vi "Control Channels2512.vi"(8 "error in (no error)":errorcluster, 10 "Values":dbl[](array[numeric]), 11 "IVI Refnum in":refnum<k15>) -> (0 "error Out":errorcluster, 3 "IVI Refnum out":refnum<k15>)   [LabVIEW 2020, in "PXI-2512 Engine.lvlib"]
uses:
  PXI-2512 Engine.lvlib
  <instrlib>/niSwitch/niSwitch.llb/niSwitch Relay Action.ctl
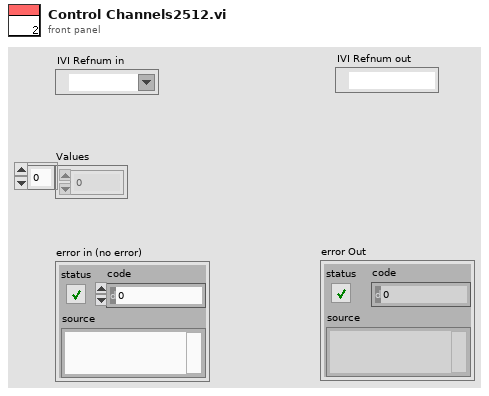
[diagram p1: front panel]
types:
  T1 = enum16{"Default", "DUT Pass Through", "DUT Open", "DUT Pass Through and FB A", "DUT Pass Through and FB B", "DUT FB A", "DUT FB B"}
  T2 = typedef "niSwitch Relay Action.ctl" = i32
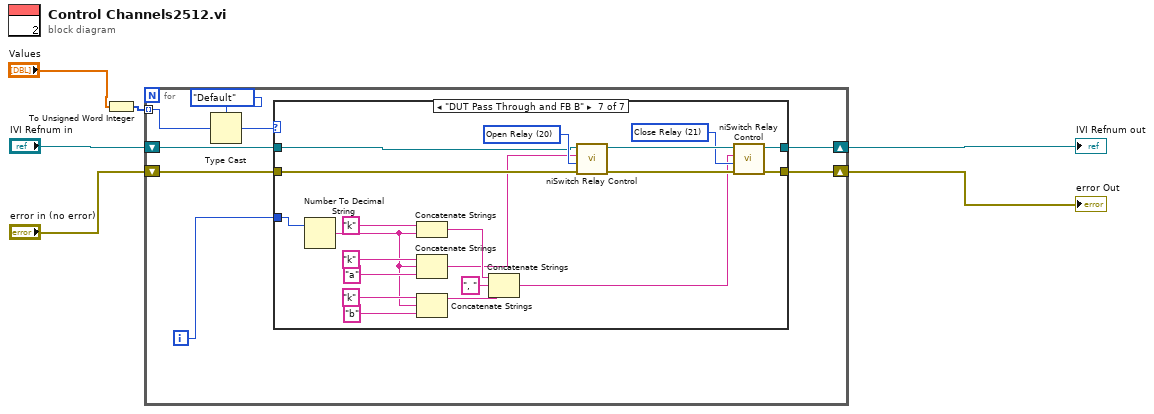
[diagram p0: block diagram]
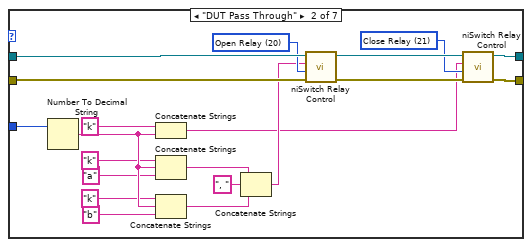
[diagram p3: hidden frame]
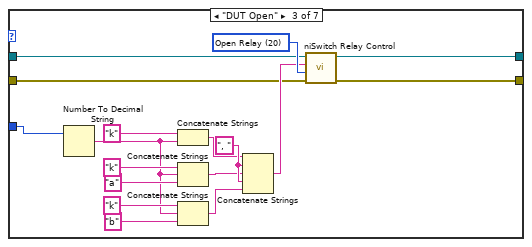
[diagram p4: hidden frame]
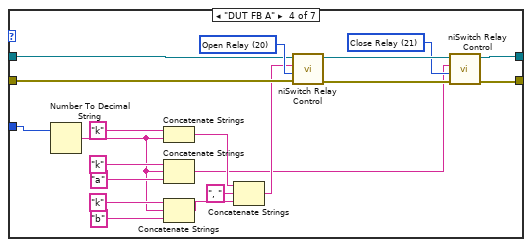
[diagram p5: hidden frame]
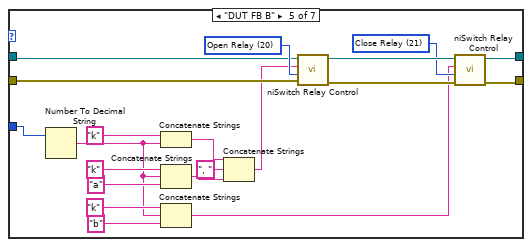
[diagram p6: hidden frame]
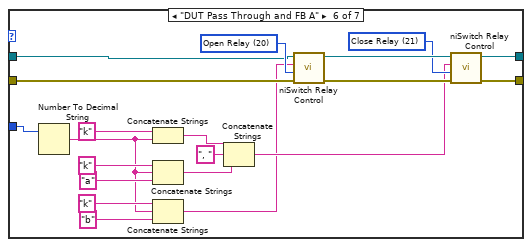
[diagram p7: hidden frame]
diagram:
  n1 = To Unsigned Word Integer(number="Values") -> (unsigned 16bit integer=w5:u16[])
  n2 = for {
    tunnel: w5 -> [w12] mode=indexing
    shift-right: [w10] -> w2
    shift-left: "IVI Refnum in" -> [w14]
    shift-right: [w8] -> w1
    shift-left: "error in (no error)" -> [w9]
    i -> [w7]
    n3 = Type Cast(type=T1."Default", x=w12) -> (*(type *) &x=w11:T1)
    n4 = case shown="\"DUT Pass Through and FB B\"" w11 {
      tunnel: w14 -> [w16 w36 w38 w61 w79 w96 w118]
      tunnel: [w16 w24 w41 w58 w77 w99 w120] -> w10
      tunnel: w9 -> [w15 w22 w37 w60 w78 w97 w117]
      tunnel: [w15 w23 w40 w59 w76 w98 w119] -> w8
      tunnel: w7 -> [_ w26 w43 w55 w84 w104 w114]
      frame "Default", Default {
      }
      frame "DUT Pass Through" {
        w19 = T2 21 items=["Open Relay"=20, "Close Relay"=21] ("relay action (Close Relay)")
        w20 = T2 20 items=["Open Relay"=20, "Close Relay"=21] ("relay action (Close Relay)")
        n5 = Number To Decimal String(number=w26) -> (decimal integer string=w34:string)  [unwired: 1 out]
        n6 = Concatenate Strings("k", w34) -> (w17:string)
        n7 = Concatenate Strings("k", w34, "a") -> (w28:string)
        n8 = Concatenate Strings("k", w34, "b") -> (w27:string)
        n9 = Concatenate Strings(w28, ", " ("string"), w27) -> (w18:string)
        n10 = call <instrlib>:"niSwitch Relay Control.vi"("error in (no error)"=w22, "relay action (Close Relay)"=w20, "relay names"=w18, "instrument handle"=w36) -> ("error out"=w21:errorcluster, "instrument handle out"=w25:refnum<k15>)  [unwired: 6 in]
        n11 = call <instrlib>:"niSwitch Relay Control.vi"("error in (no error)"=w21, "relay action (Close Relay)"=w19, "relay names"=w17, "instrument handle"=w25) -> ("error out"=w23:errorcluster, "instrument handle out"=w24:refnum<k15>)  [unwired: 6 in]
      }
      frame "DUT Open" {
        w42 = T2 20 items=["Open Relay"=20, "Close Relay"=21] ("relay action (Close Relay)")
        w53 = ", " ("string")
        n12 = Number To Decimal String(number=w43) -> (decimal integer string=w44:string)  [unwired: 1 out]
        n13 = Concatenate Strings("k", w44) -> (w47:string)
        n14 = Concatenate Strings("k", w44, "a") -> (w46:string)
        n15 = Concatenate Strings("k", w44, "b") -> (w45:string)
        n16 = Concatenate Strings(w47, w53, w46, w53, w45) -> (w39:string)
        n17 = call <instrlib>:"niSwitch Relay Control.vi"("error in (no error)"=w37, "relay action (Close Relay)"=w42, "relay names"=w39, "instrument handle"=w38) -> ("error out"=w40:errorcluster, "instrument handle out"=w41:refnum<k15>)  [unwired: 6 in]
      }
      frame "DUT FB A" {
        w62 = T2 21 items=["Open Relay"=20, "Close Relay"=21] ("relay action (Close Relay)")
        w63 = T2 20 items=["Open Relay"=20, "Close Relay"=21] ("relay action (Close Relay)")
        n18 = Number To Decimal String(number=w55) -> (decimal integer string=w68:string)  [unwired: 1 out]
        n19 = Concatenate Strings("k", w68) -> (w67:string)
        n20 = Concatenate Strings("k", w68, "a") -> (w56:string)
        n21 = Concatenate Strings("k", w68, "b") -> (w66:string)
        n22 = Concatenate Strings(w67, ", " ("string"), w66) -> (w57:string)
        n23 = call <instrlib>:"niSwitch Relay Control.vi"("error in (no error)"=w60, "relay action (Close Relay)"=w63, "relay names"=w57, "instrument handle"=w61) -> ("error out"=w64:errorcluster, "instrument handle out"=w65:refnum<k15>)  [unwired: 6 in]
        n24 = call <instrlib>:"niSwitch Relay Control.vi"("error in (no error)"=w64, "relay action (Close Relay)"=w62, "relay names"=w56, "instrument handle"=w65) -> ("error out"=w59:errorcluster, "instrument handle out"=w58:refnum<k15>)  [unwired: 6 in]
      }
      frame "DUT FB B" {
        w80 = T2 21 items=["Open Relay"=20, "Close Relay"=21] ("relay action (Close Relay)")
        w81 = T2 20 items=["Open Relay"=20, "Close Relay"=21] ("relay action (Close Relay)")
        n25 = Number To Decimal String(number=w84) -> (decimal integer string=w87:string)  [unwired: 1 out]
        n26 = Concatenate Strings("k", w87) -> (w86:string)
        n27 = Concatenate Strings("k", w87, "a") -> (w85:string)
        n28 = Concatenate Strings("k", w87, "b") -> (w74:string)
        n29 = Concatenate Strings(w86, ", " ("string"), w85) -> (w75:string)
        n30 = call <instrlib>:"niSwitch Relay Control.vi"("error in (no error)"=w78, "relay action (Close Relay)"=w81, "relay names"=w75, "instrument handle"=w79) -> ("error out"=w82:errorcluster, "instrument handle out"=w83:refnum<k15>)  [unwired: 6 in]
        n31 = call <instrlib>:"niSwitch Relay Control.vi"("error in (no error)"=w82, "relay action (Close Relay)"=w80, "relay names"=w74, "instrument handle"=w83) -> ("error out"=w76:errorcluster, "instrument handle out"=w77:refnum<k15>)  [unwired: 6 in]
      }
      frame "DUT Pass Through and FB A" {
        w100 = T2 21 items=["Open Relay"=20, "Close Relay"=21] ("relay action (Close Relay)")
        w101 = T2 20 items=["Open Relay"=20, "Close Relay"=21] ("relay action (Close Relay)")
        n32 = Number To Decimal String(number=w104) -> (decimal integer string=w107:string)  [unwired: 1 out]
        n33 = Concatenate Strings("k", w107) -> (w106:string)
        n34 = Concatenate Strings("k", w107, "a") -> (w105:string)
        n35 = Concatenate Strings("k", w107, "b") -> (w94:string)
        n36 = Concatenate Strings(w106, ", " ("string"), w105) -> (w95:string)
        n37 = call <instrlib>:"niSwitch Relay Control.vi"("error in (no error)"=w97, "relay action (Close Relay)"=w101, "relay names"=w94, "instrument handle"=w96) -> ("error out"=w102:errorcluster, "instrument handle out"=w103:refnum<k15>)  [unwired: 6 in]
        n38 = call <instrlib>:"niSwitch Relay Control.vi"("error in (no error)"=w102, "relay action (Close Relay)"=w100, "relay names"=w95, "instrument handle"=w103) -> ("error out"=w98:errorcluster, "instrument handle out"=w99:refnum<k15>)  [unwired: 6 in]
      }
      frame "DUT Pass Through and FB B" {
        w121 = T2 21 items=["Open Relay"=20, "Close Relay"=21] ("relay action (Close Relay)")
        w122 = T2 20 items=["Open Relay"=20, "Close Relay"=21] ("relay action (Close Relay)")
        n39 = Number To Decimal String(number=w114) -> (decimal integer string=w127:string)  [unwired: 1 out]
        n40 = Concatenate Strings("k", w127) -> (w126:string)
        n41 = Concatenate Strings("k", w127, "a") -> (w115:string)
        n42 = Concatenate Strings("k", w127, "b") -> (w125:string)
        n43 = Concatenate Strings(w126, ", " ("string"), w125) -> (w116:string)
        n44 = call <instrlib>:"niSwitch Relay Control.vi"("error in (no error)"=w117, "relay action (Close Relay)"=w122, "relay names"=w115, "instrument handle"=w118) -> ("error out"=w123:errorcluster, "instrument handle out"=w124:refnum<k15>)  [unwired: 6 in]
        n45 = call <instrlib>:"niSwitch Relay Control.vi"("error in (no error)"=w123, "relay action (Close Relay)"=w121, "relay names"=w116, "instrument handle"=w124) -> ("error out"=w119:errorcluster, "instrument handle out"=w120:refnum<k15>)  [unwired: 6 in]
      }
    }
  }
  "IVI Refnum out" <- w2
  "error Out" <- w1
